vi "Set Property Parameters Configuration File Required.vi"(8 "error in":errorcluster, 10 "required":bool, 11 "configuration files ref":T1 format="%.0x") -> (0 "error out":errorcluster, 3 "configuration files ref out":T1 format="%.0x")   [LabVIEW 2020, in "Ballard MIL-STD-1553 Scripting.lvlib"]
uses:
  <vilib>/NI VeriStand/Custom Device API/Custom Device Item Ref.ctl
  Constants.vi
  <vilib>/NI VeriStand/Custom Device API/Set Item Property (Boolean).vi
  Ballard MIL-STD-1553 Scripting.lvlib
  <vilib>/NI VeriStand/Custom Device API/Custom Device API.lvlib
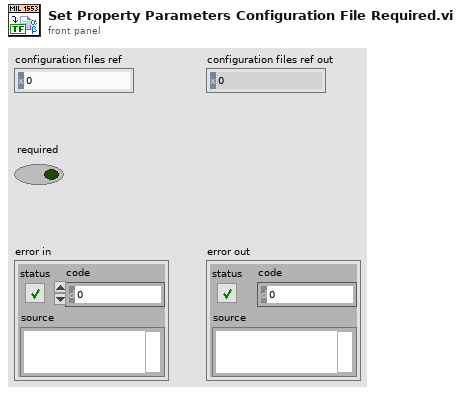
[diagram p1: front panel]
types:
  T1 = typedef "Custom Device API.lvlib/Custom Device Item Ref.ctl" = u64
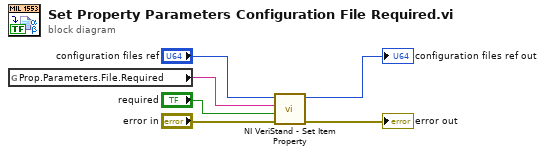
[diagram p0: block diagram]
diagram:
  n1 = global read "Constants.vi" "Prop.Parameters.File.Required"() -> (w1:string)
  n2 = call-poly <vilib>:"NI VeriStand - Set Item Property.vi"("error in (no error)"="error in", "Value"="required", "Property Name"=w1, "Item Ref in"="configuration files ref") -> ("error out"=→"error out":errorcluster, "Item Ref out"=→"configuration files ref out":T1)  [unwired: 5 in, 1 out]
